vi "run_ICov_tests.vi"(8 "error in (no error)":errorcluster, 10 "<<Unit test folder>>":path=path "C:/git/LabVIEW-knowledge-base/LabVIEW projects/DQMH Fundamentals", 11 "<<UnitTest project path>>":path=path "C:/git/LabVIEW-knowledge-base/LabVIEW projects/DQMH Fundamentals/DQMH Fundamentals - Thermal Chamber.lvproj") -> (0 "error out":errorcluster)   [LabVIEW 2018]
uses:
  <resource>/Framework/Providers/InstaCoverage/Core/Defines/TestReportTypeEnum.ctl
  <resource>/Framework/Providers/InstaCoverage/Core/InstaCoverageCore.lvlib
  <resource>/Framework/Providers/InstaCoverage/Pro/InstaCoveragePro.lvlib
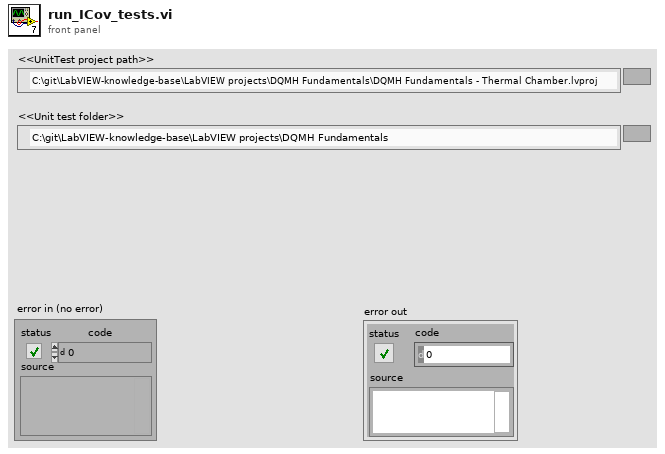
[diagram p1: front panel]
types:
  T1 = typedef "InstaCoverage.lvlib/InstaCoverageCore.lvlib/TestReportTypeEnum.ctl" = enum16{"JUNIT_XML", "HTML"}
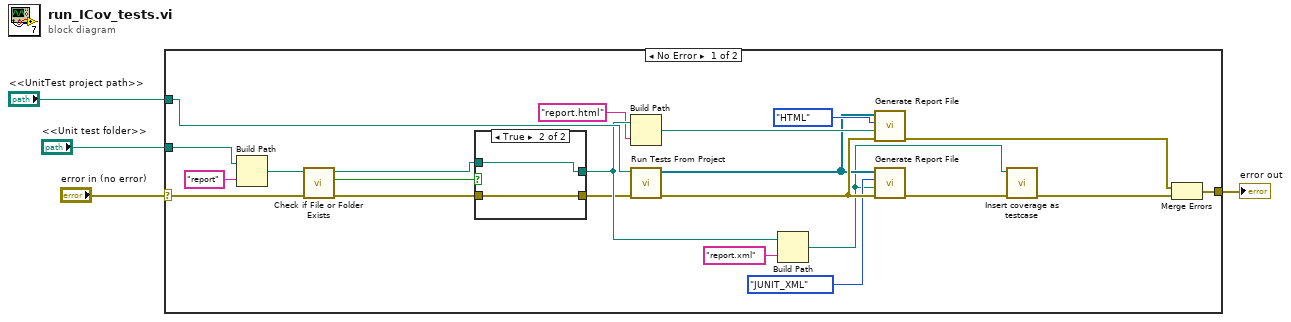
[diagram p0: block diagram]
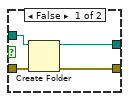
[diagram p2: hidden frame]
diagram:
  n1 = case shown="No Error" "error in (no error)" {
    selector: "error in (no error)" -> [w20 w33]
    tunnel: "<<UnitTest project path>>" -> [w18 _]
    tunnel: "<<Unit test folder>>" -> [w21 _]
    tunnel: [w9 w33] -> w1
    frame No Error {
      n2 = Build Path(base path=w21, name or relative path="report") -> (appended path=w26:path)
      n3 = call <vilib>:"Check if File or Folder Exists.vi"("error in (no error)"=w20, "path"=w26) -> ("error out"=w23:errorcluster, "file or folder exists?"=w25:bool, "dup path"=w24:path)  [unwired: 7 in]
      n4 = case shown="True" w25 {
        tunnel: w24 -> [w30 w32]
        tunnel: [w29 w32] -> w13
        tunnel: w23 -> [w28 w31]
        tunnel: [w27 w31] -> w7
        frame False {
          n5 = Create Folder(path (use dialog)=w30, error in=w28) -> (created path=w29:path, error out=w27:errorcluster)  [unwired: 1 in, 1 out]
        }
        frame True {
        }
      }
      n6 = Build Path(base path=w13, name or relative path="report.html") -> (appended path=w17:path)
      n7 = call <resource>:"Run Tests From Project.vi"("Error in"=w7, "Path lvProject"=w18) -> ("Error out"=w16:errorcluster, "TestSuite[] results"=w15:refnum<class "TestSuite.lvclass">[])  [unwired: 8 in]
      n8 = Build Path(base path=w13, name or relative path="report.xml") -> (appended path=w8:path)
      n9 = call <resource>:"Generate Report File.vi"("Error In"=w16, "Path reportFile"=w17, "TestReportTypeEnum in"=TestReportTypeEnum."HTML", "TestSuite[] in"=w15) -> ("Error Out"=w5:errorcluster)  [unwired: 7 in]
      n10 = call <resource>:"Generate Report File.vi"("Error In"=w16, "Path reportFile"=w8, "TestReportTypeEnum in"=TestReportTypeEnum."JUNIT_XML", "TestSuite[] in"=w15) -> ("Error Out"=w6:errorcluster)  [unwired: 7 in]
      n11 = call "Insert coverage as testcase.vi"("Error in"=w6, "Path instaCoverageReport"=w8) -> ("error out"=w10:errorcluster)  [unwired: 9 in]
      n12 = Merge Errors(w5, w10) -> (w9:errorcluster)
    }
    frame Error {
    }
  }
  "error out" <- w1
